vi "Acquisition.vi"() -> ()   [LabVIEW 2018]
uses:
  Type/_Run State.ctl
  Type/_File Type.ctl
  Type/_RT Command.ctl
  Type/_Data Operation.ctl
  Type/_Run Module.ctl
  Configuration/_Global Configuration.vi
  <vilib>/Utility/config.llb/Read Key (Path).vi
  <vilib>/Utility/config.llb/Read Key (String).vi
  <vilib>/Utility/config.llb/Write Key (Path).vi
  <vilib>/Utility/config.llb/Write Key (String).vi
  <vilib>/Utility/file.llb/Read From Spreadsheet File (string).vi
  <vilib>/Utility/miscctls.llb/LVRectTypeDef.ctl
  <vilib>/Utility/config.llb/NI_LVConfig.lvlib
panel:
  in  "Equilibration Time":u32
  in  "Editor":bool
  out "# of Samp":i32=1 caption="# of Samples"
  in  "Sample Description":string
  in  "Sync Mode":enum32{"Manual", "LC Sync"}(radio)
  in  "Data Folder":path
  in  "Save":bool
  in  "Load":bool
  in  "Insert":bool
  in  "Delete":bool
  in  "Import":bool
  in  "Export":bool
  in  "Sample List":i32(listbox)
  in  "Run":bool
  in  "Cancel":bool
  in  "List File":path
  out "Run Time":i32=1 caption="Run Time (ms)"
  in  "Current Sample":i32=1 min=0
  in  "Method File":path
  # "(mS)"
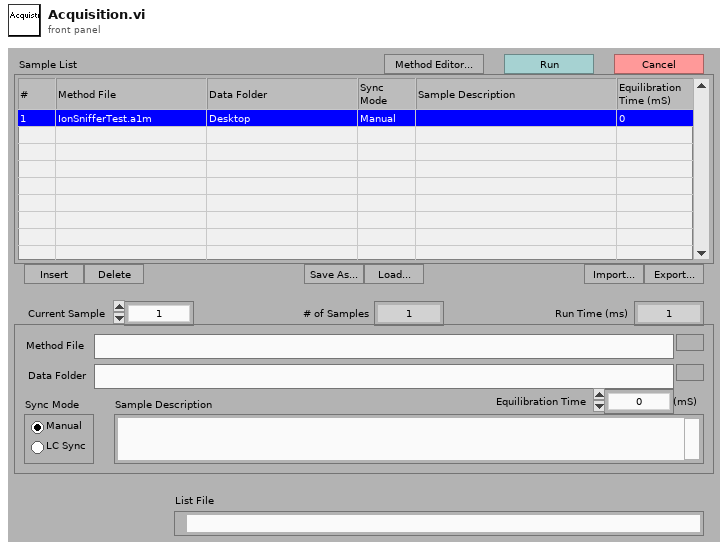
[diagram p1: front panel]
types:
  T1 = typedef "_Run State.ctl" = enum16{"Init", "Update", "Start", "End", "Error"}
  T2 = typedef "_File Type.ctl" = enum16{"Configuration", "Old Configuration", "Calibration", "Resolution", "Diagnostic Method", "Old Method", "Acq Method", "Samp List"}
  T3 = typedef "LVRectTypeDef.ctl" = cluster{"Left":i16, "Top":i16, "Right":i16, "Bottom":i16}
  T4 = typedef "_RT Command.ctl" = enum16{"xml Start Run", "xml Start Actual Run", "xml Stop Run", "xml Runtime Update", "xml Get Status", "xml Get Table", "xml Set Table", "xml Get Configuration", "xml System Status", "xml Set LC Input Logic", "xml Get Data", "xml Get Info", "Start", "StartActualRun", "Stop", "Runtime Update", "Get Data", "Get Info", "Get Status", "Get Param", "Get Config", "Get Table", "Read ADC", "Set Oscillator", "Update Config", "Update Table", "Set All Pol", "Set Pol and DC", "Set Max Mass", "Toggle RP", "Toggle EL", "Set PIC", "Initialize Turbo", "Send Turbo Comm", "Close Turbo", "P1", "P2", "P3", "Send Serial", "Set LC Out", "Get LC In", "Read VAC", "Test Table", "Toggle Power", "Get Startup", "Set Startup", "Get ADC Table", "Set ADC Table", "Get Brief Status", "Get Detail Status", "Auxiliary Update", "Set CC Logics", "Set CC Input Logics", "Ignore Error", "invalid"}
  T5 = typedef "_Data Operation.ctl" = enum8{"Initialize", "Get Data", "Set Data", "Close"}
  T6 = enum32{"Bad", "Idle", "Run top level", "Running"}
  T7 = enum32{"existing file", "new file", "new or existing file", "existing dir", "new dir", "new or existing dir", "existing file (use LLBs)", "new file (use LLBs)", "new or existing file (use LLBs)", "new or existing file or directory (use LLBs)"}
  T8 = typedef "NI_LVConfig.lvlib/Config Data RefNum.ctl" = refnum<k1>
  T9 = cluster{"Update":bool, "Running":bool, "List File":path, "Sample List":string[][]}
  T10 = typedef "_Run Module.ctl" = u16
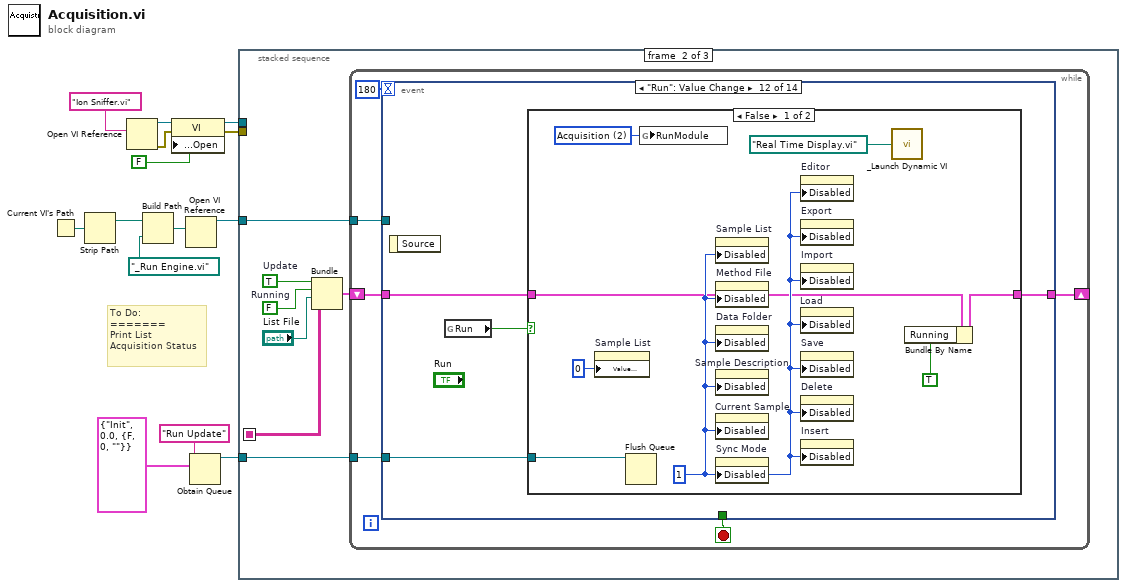
[diagram p0: block diagram]
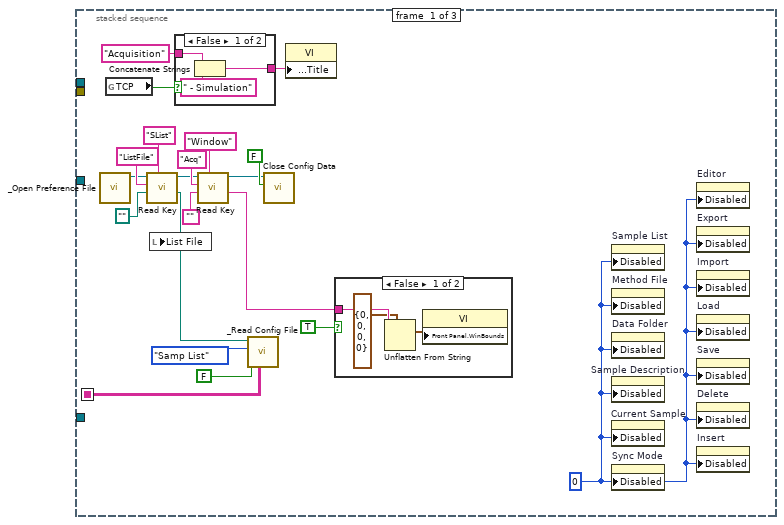
[diagram p2: hidden frame]
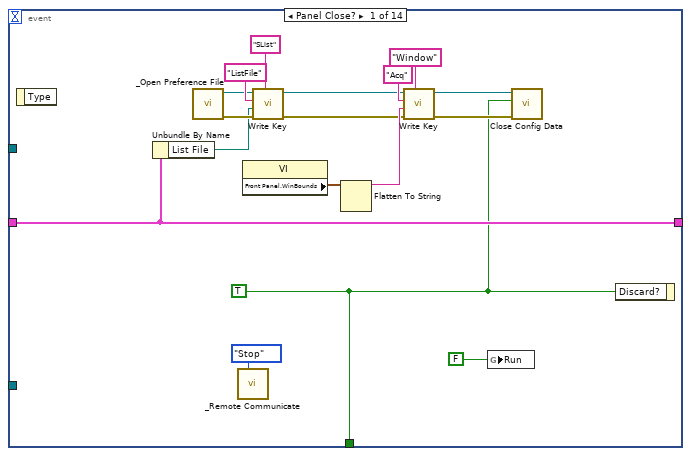
[diagram p5: hidden frame]
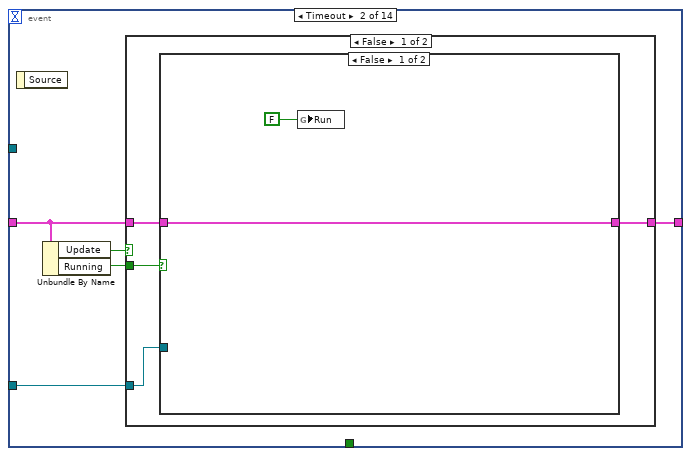
[diagram p6: hidden frame]
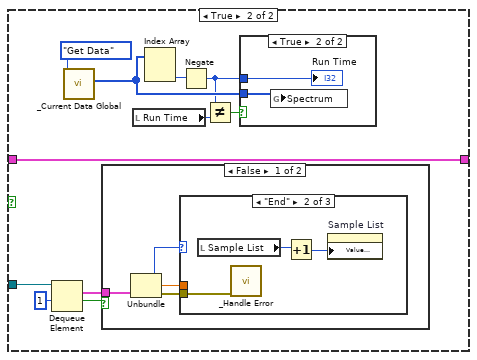
[diagram p7: hidden frame]
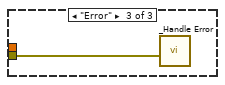
[diagram p10: hidden frame]
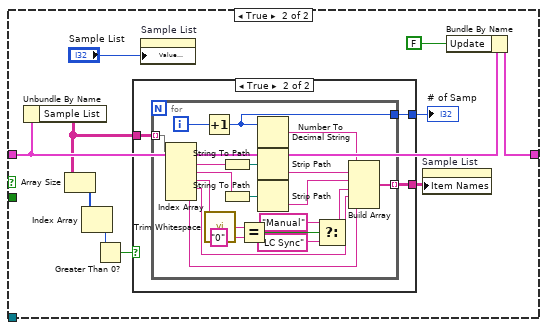
[diagram p12: hidden frame]
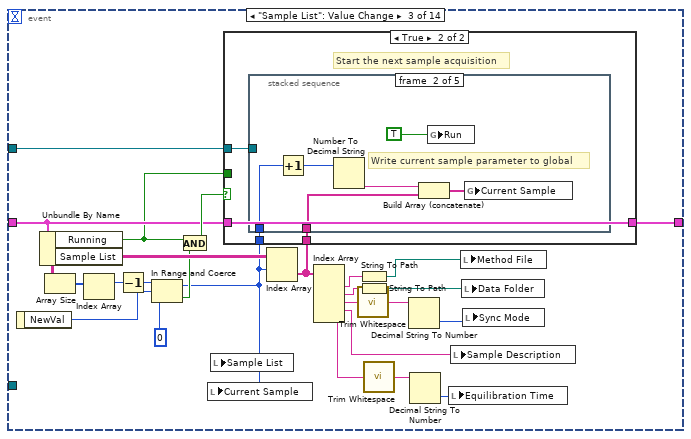
[diagram p14: hidden frame]
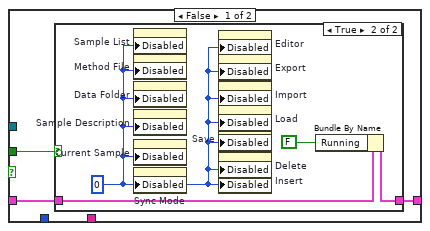
[diagram p15: hidden frame]
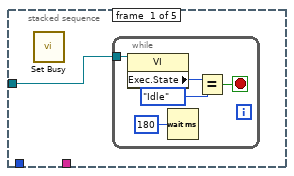
[diagram p17: hidden frame]
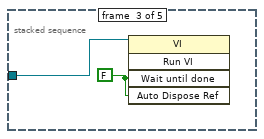
[diagram p18: hidden frame]
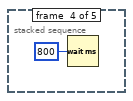
[diagram p19: hidden frame]
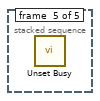
[diagram p20: hidden frame]
diagram:
  # "To Do:\n=======\nPrint List\nAcquisition Status"
  n1 = Current VI's Path() -> (path=w11:path)
  n2 = Strip Path(path=w11) -> (stripped path=w7:path)  [unwired: 1 out]
  n3 = Open VI Reference(vi path="Ion Sniffer.vi") -> (vi reference=w5:refnum<vi>, error out=w4:errorcluster)  [unwired: 1 in, 4 out]
  n4 = Build Path(base path=w7, name or relative path=path "_Run Engine.vi") -> (appended path=w9:path)
  n5 = property class="VI"(reference=w5, error in=w4, "Front Panel Window:Open"=FALSE) -> (reference out=w2:refnum<vi>, error out=w1:errorcluster)
  n6 = Open VI Reference(vi path=w9) -> (vi reference=w8:refnum<vi>)  [unwired: 1 in, 5 out]
  n7 = Obtain Queue(name (unnamed)="Run Update", element data type=cluster{T1, dbl, "error out":errorcluster} {enum."Init", 0.0, "error out"={"status"=FALSE, "code"=0, "source"=""}}) -> (queue out=w12:refnum<queue>)  [unwired: 3 in, 2 out]
  n8 = stacked-sequence {
    seq-local: [w17 _ _] -> [_ w42 _]
    tunnel: w12 -> [_ w48 w344]
    tunnel: w8 -> [_ w47 w343]
    tunnel: w2 -> [_ _ w339]
    tunnel: w1 -> [_ _ w338]
    frame #0 {
      w16 = u8 0 ("Disabled")
      n9 = call "_Open Preference File.vi"() -> ("refnum"=w22:T8)  [unwired: 3 in, 4 out]
      n10 = global read "_Global Configuration.vi" "TCP"() -> (w32:bool)
      n11 = call-poly <vilib>:"Read Key.vi"("section"="SList", "default value"=path "", "key"="ListFile", "refnum"=w22) -> ("value"=w18:path, "refnum out"=w23:T8)  [unwired: 1 in, 5 out]
      n12 = local write "List File"(w18) -> ()
      n13 = case shown="False" w32 {
        tunnel: "Acquisition" ("string") -> [w40 w41]
        tunnel: [w38 w41] -> w33
        frame False {
          n14 = Concatenate Strings(w40, " - Simulation" ("string")) -> (w38:string)
        }
        frame True {
        }
      }
      n15 = call-poly <vilib>:"Read Key.vi"("section"="Window", "default value"="", "key"="Acq" ("section"), "refnum"=w23) -> ("value"=w25:string, "refnum out"=w21:T8)  [unwired: 2 in, 4 out]
      n16 = call "_Read Config File.vi"("advisory dialog? (display:T)"=FALSE, "File Type (config)"=_File_Type."Samp List", "start path  (Not A Path)"=w18) -> ("Sample List"=w17:string[][])  [unwired: 8 out]
      n17 = call <vilib>:"Close Config Data.vi"("write file if changed (T)"=FALSE ("write configuration file? (F)"), "refnum"=w21) -> ()  [unwired: 1 in, 9 out]
      n18 = property class="VI"("Front Panel Window:Title"=w33) -> ()  [unwired: 2 in, 2 out]
      n19 = case shown="False" TRUE {
        tunnel: w25 -> [w37 _]
        frame False {
          n20 = Unflatten From String(type=T3 {"Left"=0, "Top"=0, "Right"=0, "Bottom"=0} ("Front Panel Window:Window Bounds"), binary string=w37) -> (value=w35:T3)  [unwired: 1 in, 4 out]
          n21 = property class="VI"("Front Panel.WinBounds"=w35) -> ()  [unwired: 2 in, 2 out]
        }
        frame True {
        }
      }
      n22 = property on="Sample List" class="MCListbox (strict)"("Disabled"=w16) -> ()  [unwired: 2 in, 2 out]
      n23 = property on="Method File" class="Path"("Disabled"=w16) -> ()  [unwired: 2 in, 2 out]
      n24 = property on="Data Folder" class="Path"("Disabled"=w16) -> ()  [unwired: 2 in, 2 out]
      n25 = property on="Sample Description" class="Str"("Disabled"=w16) -> ()  [unwired: 2 in, 2 out]
      n26 = property on="Current Sample" class="DigNum (strict)"("Disabled"=w16) -> ()  [unwired: 2 in, 2 out]
      n27 = property on="Sync Mode" class="RadioBtnsControl (strict)"("Disabled"=w16) -> ()  [unwired: 2 in, 2 out]
      n28 = property on="Editor" class="Bool"("Disabled"=w16) -> ()  [unwired: 2 in, 2 out]
      n29 = property on="Export" class="Bool"("Disabled"=w16) -> ()  [unwired: 2 in, 2 out]
      n30 = property on="Import" class="Bool"("Disabled"=w16) -> ()  [unwired: 2 in, 2 out]
      n31 = property on="Load" class="Bool"("Disabled"=w16) -> ()  [unwired: 2 in, 2 out]
      n32 = property on="Save" class="Bool"("Disabled"=w16) -> ()  [unwired: 2 in, 2 out]
      n33 = property on="Delete" class="Bool"("Disabled"=w16) -> ()  [unwired: 2 in, 2 out]
      n34 = property on="Insert" class="Bool"("Disabled"=w16) -> ()  [unwired: 2 in, 2 out]
    }
    frame #1 {
      w45 = FALSE  # Running
      w46 = TRUE  # Update
      n35 = Bundle("Update"=w46, "Running"=w45, "List File"="List File", "Sample List"=w42) -> (w44:T9)  [unwired: 1 out]
      n36 = while {
        shift-right: [w51] -> _
        shift-left: w44 -> [w53]
        tunnel: w48 -> [w50]
        tunnel: w47 -> [w49]
        stop <- w54 stop-if-true
        n37 = event shown="[11] \"Run\": Value Change" {
          selector: _ -> [_ _ _ _ _ _ _ _ _ _ _ _ _ _]
          dyn-events: _ -> [_ _ _ _ _ _ _ _ _ _ _ _ _ _]
          timeout: 180 -> [_ _ _ _ _ _ _ _ _ _ _ _ _ _]
          tunnel: [w55 _ _ _ _ _ _ _ _ _ _ _ _ _] -> w54
          tunnel: w53 -> [w66 w74 w144 w190 w206 w219 w227 w241 w249 w269 w305 w309 w325 w337]
          tunnel: [w66 w76 w143 w190 w205 w217 w225 w239 w248 w269 w307 w310 w321 w337] -> w51
          tunnel: w50 -> [_ w75 _ _ _ _ _ _ _ _ _ w311 _ _]
          tunnel: w49 -> [_ _ w145 _ _ _ _ _ _ _ _ _ w324 _]
          event Panel Close? {
            w55 = TRUE ("Discard?")
            n38 = event-data() -> ()  [unwired: 2 out]
            n39 = Unbundle By Name(w66) -> ("List File"=w65:path)
            n40 = call "_Open Preference File.vi"() -> ("error"=w68:errorcluster, "refnum"=w69:T8)  [unwired: 3 in, 3 out]
            n41 = call "_Remote Communicate.vi"("Command"=_RT_Command."Stop") -> ()  [unwired: 5 in, 4 out]
            n42 = property class="VI"() -> ("Front Panel.WinBounds"=w63:T3)  [unwired: 2 in, 2 out]
            n43 = call-poly <vilib>:"Write Key.vi"("section"="SList", "error in (no error)"=w68, "value"=w65, "key"="ListFile", "refnum"=w69) -> ("error out"=w56:errorcluster, "refnum out"=w57:T8)  [unwired: 5 out]
            n44 = Flatten To String(anything=w63) -> (data string=w62:string)  [unwired: 1 in, 4 out]
            n45 = call-poly <vilib>:"Write Key.vi"("section"="Window", "error in (no error)"=w56, "value"=w62, "key"="Acq" ("section"), "refnum"=w57) -> ("error out"=w58:errorcluster, "refnum out"=w59:T8)  [unwired: 1 in, 4 out]
            n46 = global write "_Global Configuration.vi" "Run"(FALSE ("Update")) -> ()
            n47 = call <vilib>:"Close Config Data.vi"("error in (no error)"=w58, "write file if changed (T)"=w55, "refnum"=w59) -> ()  [unwired: 9 out]
            n48 = event-data("Discard?"=w55) -> ()  [unwired: 1 in, 1 out]
          }
          event Timeout {
            n49 = event-data() -> ()  [unwired: 2 out]
            n50 = Unbundle By Name(w74) -> ("Update"=w73:bool, "Running"=w72:bool)
            n51 = case shown="False" w73 {
              tunnel: w74 -> [w78 w113]
              tunnel: [w77 w111] -> w76
              tunnel: w72 -> [w80 _]
              tunnel: w75 -> [w79 _]
              frame False {
                n52 = case shown="False" w80 {
                  tunnel: w79 -> [_ w93]
                  tunnel: w78 -> [w82 w83]
                  tunnel: [w82 w83] -> w77
                  frame False {
                    n53 = global write "_Global Configuration.vi" "Run"(FALSE ("Update")) -> ()
                  }
                  frame True {
                    n54 = Dequeue Element(queue=w93, timeout in ms (-1)=1) -> (element=w91:cluster{T1, dbl, "error out":errorcluster}, timed out?=w90:bool)  [unwired: 1 in, 2 out]
                    n55 = call "_Current Data Global.vi"("Operation"=_Data_Operation."Get Data") -> ("Latest Raw Data"=w86:i32[])  [unwired: 3 in, 3 out]
                    n56 = case shown="False" w90 {
                      tunnel: w91 -> [w99 _]
                      frame False {
                        n57 = Unbundle(w99) -> (w98:T1, w96:dbl, "error out"=w97:errorcluster)
                        n58 = case shown="\"End\"" w98 {
                          tunnel: w97 -> [_ w102 w103]
                          tunnel: w96 -> [_ _ _]
                          frame "Init", Default {
                          }
                          frame "End" {
                            n59 = local read "Sample List"() -> (w101:i32)
                            n60 = call "_Handle Error.vi"("error in (no error)"=w102) -> ()  [unwired: 2 in, 5 out]
                            n61 = Increment(x=w101) -> (x+1=w100:i32)
                            n62 = property on="Sample List" class="MCListbox (strict)"("Value (Signaling)"=w100) -> ()  [unwired: 2 in, 2 out]
                          }
                          frame "Error" {
                            n63 = call "_Handle Error.vi"("error in (no error)"=w103) -> ()  [unwired: 2 in, 5 out]
                          }
                        }
                      }
                      frame True {
                      }
                    }
                    n64 = local read "Run Time"() -> (w88:i32)
                    n65 = Index Array(array=w86) -> (element #2=w85:i32)  [unwired: 2 in, 1 out]
                    n66 = Negate(x=w85) -> (-x=w84:i32)
                    n67 = Not Equal?(x=w84, y=w88) -> (x != y?=w87:bool)
                    n68 = case shown="True" w87 {
                      tunnel: w86 -> [_ w94]
                      tunnel: w84 -> [_ w95]
                      frame False {
                      }
                      frame True {
                        n69 = global write "_Global Configuration.vi" "Spectrum"(w94) -> ()
                        "Run Time" <- w95
                      }
                    }
                  }
                }
              }
              frame True {
                n70 = Unbundle By Name(w113) -> ("Sample List"=w107:string[][])
                n71 = Array Size(array=w107) -> (size(s)=w106:i32[])
                n72 = Index Array(array=w106) -> (element=w105:i32)  [unwired: 1 in]
                n73 = Greater Than 0?(x=w105) -> (x > 0?=w104:bool)
                n74 = case shown="True" w104 {
                  tunnel: [_ w116] -> w109
                  tunnel: [_ w115] -> w108
                  tunnel: w107 -> [_ w114]
                  frame False {
                  }
                  frame True {
                    n75 = for {
                      tunnel: w114 -> [w136] mode=indexing
                      tunnel: [w134] -> w116
                      tunnel: [w119] -> w115 mode=indexing
                      i -> [w135]
                      n76 = Index Array(array=w136) -> (element #1=w133:string, element #2=w130:string, element #3=w129:string, element #4=w120:string, element #5=w117:string)  [unwired: 5 in]
                      n77 = Increment(x=w135) -> (x+1=w134:i32)
                      n78 = call <vilib>:"Trim Whitespace.vi"("string"=w129) -> ("trimmed string"=w127:string)  [unwired: 1 in]
                      n79 = String To Path(string=w133) -> (path=w132:path)
                      n80 = String To Path(string=w130) -> (path=w131:path)
                      n81 = Equal?(x=w127, y="0") -> (x = y?=w128:bool)
                      n82 = Number To Decimal String(number=w134) -> (decimal integer string=w124:string)  [unwired: 1 out]
                      n83 = Strip Path(path=w132) -> (name=w123:string)  [unwired: 1 out]
                      n84 = Strip Path(path=w131) -> (name=w122:string)  [unwired: 1 out]
                      n85 = Select(t="Manual" ("y"), s=w128, f="LC Sync" ("y")) -> (s? t:f=w121:string)
                      n86 = Build Array(w124, w123, w122, w121, w120, w117) -> (w119:string[])
                    }
                  }
                }
                "# of Samp" <- w109
                n87 = property on="Sample List" class="MCListbox (strict)"("Value (Signaling)"="Sample List") -> ()  [unwired: 2 in, 2 out]
                n88 = property on="Sample List" class="MCListbox (strict)"("Item Names"=w108) -> ()  [unwired: 2 in, 2 out]
                n89 = Bundle By Name(cluster=w113, "Update"=FALSE) -> (w111:T9)
              }
            }
          }
          event "Sample List": Value Change {
            n90 = event-data() -> ("NewVal"=w161:i32)  [unwired: 1 out]
            n91 = Unbundle By Name(w144) -> ("Running"=w142:bool, "Sample List"=w158:string[][])
            n92 = Array Size(array=w158) -> (size(s)=w156:i32[])
            n93 = Index Array(array=w156) -> (element=w157:i32)  [unwired: 1 in]
            n94 = Decrement(x=w157) -> (x-1=w159:i32)
            n95 = In Range and Coerce(upper limit=w159, x=w161, lower limit=0) -> (coerced(x)=w140:i32, In Range?=w147:bool)
            n96 = And(x=w142, y=w147) -> (x .and. y?=w146:bool)
            n97 = local write "Current Sample"(w140) -> ()
            n98 = local write "Sample List"(w140) -> ()
            n99 = Index Array(array=w158, index (row)=w140) -> (element=w141:string[])  [unwired: 1 in]
            n100 = case shown="True" w146 {
              tunnel: w145 -> [_ w173]
              tunnel: w144 -> [w164 w172]
              tunnel: [w163 w172] -> w143
              tunnel: w142 -> [w162 _]
              tunnel: w141 -> [_ w171]
              tunnel: w140 -> [_ w170]
              frame False {
                n101 = case shown="True" w162 {
                  tunnel: w164 -> [w165 w169]
                  tunnel: [w165 w168] -> w163
                  frame False {
                  }
                  frame True {
                    w167 = u8 0 ("Disabled")
                    n102 = property on="Sample List" class="MCListbox (strict)"("Disabled"=w167) -> ()  [unwired: 2 in, 2 out]
                    n103 = property on="Method File" class="Path"("Disabled"=w167) -> ()  [unwired: 2 in, 2 out]
                    n104 = property on="Data Folder" class="Path"("Disabled"=w167) -> ()  [unwired: 2 in, 2 out]
                    n105 = property on="Sample Description" class="Str"("Disabled"=w167) -> ()  [unwired: 2 in, 2 out]
                    n106 = property on="Current Sample" class="DigNum (strict)"("Disabled"=w167) -> ()  [unwired: 2 in, 2 out]
                    n107 = property on="Sync Mode" class="RadioBtnsControl (strict)"("Disabled"=w167) -> ()  [unwired: 2 in, 2 out]
                    n108 = property on="Editor" class="Bool"("Disabled"=w167) -> ()  [unwired: 2 in, 2 out]
                    n109 = property on="Export" class="Bool"("Disabled"=w167) -> ()  [unwired: 2 in, 2 out]
                    n110 = property on="Import" class="Bool"("Disabled"=w167) -> ()  [unwired: 2 in, 2 out]
                    n111 = property on="Load" class="Bool"("Disabled"=w167) -> ()  [unwired: 2 in, 2 out]
                    n112 = property on="Save" class="Bool"("Disabled"=w167) -> ()  [unwired: 2 in, 2 out]
                    n113 = property on="Delete" class="Bool"("Disabled"=w167) -> ()  [unwired: 2 in, 2 out]
                    n114 = property on="Insert" class="Bool"("Disabled"=w167) -> ()  [unwired: 2 in, 2 out]
                    n115 = Bundle By Name(cluster=w169, "Running"=FALSE) -> (w168:T9)
                  }
                }
              }
              frame True {
                # "Start the next sample acquisition"
                n116 = stacked-sequence {
                  tunnel: w173 -> [w174 _ w186 _ _]
                  tunnel: w171 -> [_ w184 _ _ _]
                  tunnel: w170 -> [_ w181 _ _ _]
                  frame #0 {
                    n117 = call <vilib>:"Set Busy.vi"() -> ()  [unwired: 4 in, 8 out]
                    n118 = while {
                      tunnel: w174 -> [w179]
                      stop <- w176 stop-if-true
                      n119 = property class="VI"(reference=w179) -> ("Exec.State"=w178:T6)  [unwired: 1 in, 2 out]
                      n120 = Wait (ms)(milliseconds to wait=u32 180) -> ()  [unwired: 1 out]
                      n121 = Equal?(x=w178, y=T6."Idle") -> (x = y?=w176:bool)
                    }
                  }
                  frame #1 {
                    # "Write current sample parameter to global"
                    n122 = Increment(x=w181) -> (x+1=w180:i32)
                    n123 = Number To Decimal String(number=w180) -> (decimal integer string=w182:string)  [unwired: 1 out]
                    n124 = Build Array (concatenate)(w182, w184) -> (w183:string[])
                    n125 = global write "_Global Configuration.vi" "Run"(TRUE ("Update")) -> ()
                    n126 = global write "_Global Configuration.vi" "Current Sample"(w183) -> ()
                  }
                  frame #2 {
                    w187 = FALSE ("Wait until done")
                    n127 = invoke class="VI" method="Run VI"(reference=w186, "Wait until done"=w187, "Auto Dispose Ref"=w187) -> ()  [unwired: 2 in, 5 out]
                  }
                  frame #3 {
                    n128 = Wait (ms)(milliseconds to wait=u32 800) -> ()  [unwired: 1 out]
                  }
                  frame #4 {
                    n129 = call <vilib>:"Unset Busy.vi"() -> ()  [unwired: 2 in, 10 out]
                  }
                }
              }
            }
            n130 = Index Array(array=w141) -> (element #1=w152:string, element #2=w153:string, element #3=w154:string, element #4=w155:string, element #5=w138:string)  [unwired: 5 in]
            n131 = call <vilib>:"Trim Whitespace.vi"("string"=w154) -> ("trimmed string"=w149:string)  [unwired: 1 in]
            n132 = String To Path(string=w152) -> (path=w151:path)
            n133 = String To Path(string=w153) -> (path=w150:path)
            n134 = call <vilib>:"Trim Whitespace.vi"("string"=w138) -> ("trimmed string"=w139:string)  [unwired: 1 in]
            n135 = Decimal String To Number(string=w149) -> (number=w148:i32)  [unwired: 3 out]
            n136 = Decimal String To Number(string=w139) -> (number=w137:i32)  [unwired: 3 out]
            n137 = local write "Equilibration Time"(w137) -> ()
            n138 = local write "Sample Description"(w155) -> ()
            n139 = local write "Method File"(w151) -> ()
            n140 = local write "Data Folder"(w150) -> ()
            n141 = local write "Sync Mode"(w148) -> ()
          }
          event "Current Sample": Value Change {
            n142 = event-data() -> ("NewVal"=w189:i32)  [unwired: 1 out]
            n143 = property on="Sample List" class="MCListbox (strict)"("Value (Signaling)"=w189) -> ()  [unwired: 2 in, 2 out]
          }
          event "Insert": Value Change {
            n144 = event-data() -> ()  [unwired: 2 out]
            n145 = call "Please enter # of samples to insert."() -> ("# of Samples to Insert"=w203:dbl)  [unwired: 2 in, 17 out]
            n146 = Unbundle By Name(w206) -> ("Sample List"=w198:string[][])
            n147 = local read "Sample List"() -> (w197:i32)
            n148 = To Long Integer(number=w203) -> (32bit integer=w202:i32)
            n149 = In Range and Coerce(upper limit=2147483647, x=w202, lower limit=1) -> (coerced(x)=w199:i32)  [unwired: 1 out]
            n150 = Index Array(array=w198, index (row)=w197) -> (element=w193:string[])  [unwired: 1 in]
            n151 = Array Size(array=w193) -> (size(s)=w195:i32)
            n152 = Greater Than 0?(x=w195) -> (x > 0?=w194:bool)
            n153 = Select(t=w193, s=w194, f=string[] ["", "", "1", "", "0"] ("appended array")) -> (s? t:f=w191:string[])
            n154 = for {
              N: w199 -> [_]
              shift-right: [w208] -> w196
              shift-left: w198 -> [w210]
              tunnel: w197 -> [w209]
              tunnel: w191 -> [w207]
              n155 = Insert Into Array(array=w210, index (row)=w209, new element=w207) -> (w208:string[][])  [unwired: 1 in]
            }
            n156 = Bundle By Name(cluster=w206, "Sample List"=w196, "Update"=TRUE) -> (w205:T9)
          }
          event "Delete": Value Change {
            n157 = event-data() -> ()  [unwired: 2 out]
            n158 = Unbundle By Name(w219) -> ("Sample List"=w218:string[][])
            n159 = Two Button Dialog(message="Please choose a delete option.", 1:"Delete All Samples" ("T button name (\"OK\")"), 2:"Delete Current Sample" ("T button name (\"OK\")")) -> (T button?=w211:bool)
            n160 = case shown="True" w211 {
              tunnel: w218 -> [_ w223]
              tunnel: [_ w220] -> w216
              frame False {
              }
              frame True {
                n161 = local read "Sample List"() -> (w221:i32)
                n162 = Delete From Array(array=w223, length=1, index (row)=w221) -> (array with subset deleted=w220:string[][])  [unwired: 1 in, 1 out]
              }
            }
            n163 = Bundle By Name(cluster=w219, "Sample List"=w216, "Update"=TRUE) -> (w217:T9)
          }
          event "Save": Value Change {
            n164 = event-data() -> ()  [unwired: 2 out]
            n165 = Unbundle By Name(w227) -> ("List File"=w229:path, "Sample List"=w228:string[][])
            n166 = call "_Save Config File.vi"("Sample List"=w228, "File Type (config)"=_File_Type."Samp List", "start path  (Not A Path)"=w229) -> ("error"=w226:bool, "new file path"=w224:path)  [unwired: 5 in, 2 out]
            n167 = case shown="False" w226 {
              tunnel: w227 -> [w233 w234]
              tunnel: [w232 w234] -> w225
              tunnel: w224 -> [w231 _]
              frame False {
                n168 = local write "List File"(w231) -> ()
                n169 = Bundle By Name(cluster=w233, "List File"=w231) -> (w232:T9)
              }
              frame True {
              }
            }
          }
          event "Load": Value Change {
            n170 = event-data() -> ()  [unwired: 2 out]
            n171 = Unbundle By Name(w241) -> ("List File"=w238:path)
            n172 = call "_Read Config File.vi"("File Type (config)"=_File_Type."Samp List", "start path  (Not A Path)"=w238) -> ("error"=w240:bool, "new file path"=w235:path, "Sample List"=w236:string[][])  [unwired: 3 in, 4 out]
            n173 = case shown="False" w240 {
              tunnel: w241 -> [w246 w247]
              tunnel: [w245 w247] -> w239
              tunnel: w235 -> [w244 _]
              tunnel: w236 -> [w242 _]
              frame False {
                n174 = Bundle By Name(cluster=w246, "Update"=TRUE, "Sample List"=w242, "List File"=w244) -> (w245:T9)
                n175 = local write "List File"(w244) -> ()
              }
              frame True {
              }
            }
          }
          event "Import": Value Change {
            n176 = event-data() -> ()  [unwired: 2 out]
            n177 = Unbundle By Name(w249) -> ("List File"=w252:path)
            n178 = call "_Get File.vi"("For Write (T)"=FALSE, "select mode (new or existing)"=T7."existing file", "extension (isd)"="*.txt" ("pattern (all files)"), "prompt"="Please select a sample list import file.", "Start Path"=w252) -> ("Seleted File"=w250:path, "Exists"=w258:bool, "Succeeded"=w257:bool)  [unwired: 1 in, 1 out]
            n179 = And(x=w257, y=w258) -> (x .and. y?=w251:bool)
            n180 = case shown="True" w251 {
              tunnel: w250 -> [_ w264]
              tunnel: w249 -> [w259 w263]
              tunnel: [w259 w262] -> w248
              frame False {
              }
              frame True {
                n181 = call-poly <vilib>:"Read From Spreadsheet File.vi"("file path (dialog if empty)"=w264) -> ("all rows"=w266:string[][])  [unwired: 3 in, 7 out]
                n182 = Delete From Array(array=w266, length=1, index (row)=0) -> (array with subset deleted=w261:string[][])  [unwired: 1 in, 1 out]
                n183 = Bundle By Name(cluster=w263, "Update"=TRUE, "Sample List"=w261) -> (w262:T9)
              }
            }
          }
          event "Export": Value Change {
            n184 = event-data() -> ()  [unwired: 2 out]
            n185 = Unbundle By Name(w269) -> ("Sample List"=w270:string[][], "List File"=w277:path)
            n186 = property on="Sample List" class="MCListbox (strict)"() -> ("ColHdrString"=w274:string[])  [unwired: 2 in, 2 out]
            n187 = call "_Get File.vi"("For Write (T)"=TRUE, "select mode (new or existing)"=T7."new or existing file", "default name"="My Sample List", "extension (isd)"="*.txt" ("pattern (all files)"), "prompt"="Please enter a sample list export file name.", "Start Path"=w277) -> ("Seleted File"=w276:path, "Succeeded"=w275:bool)  [unwired: 2 out]
            n188 = Delete From Array(array=w274, length=1, index=0) -> (array with subset deleted=w271:string[])  [unwired: 1 out]
            n189 = case shown="True" w275 {
              tunnel: w276 -> [_ w283]
              tunnel: w271 -> [_ w285]
              tunnel: w270 -> [_ w284]
              frame False {
              }
              frame True {
                n190 = Build Array (concatenate)(w285, w284) -> (w282:string[][])
                n191 = call "_Export Table To Text File.vi"("2D data"=w282, "file path (dialog if empty)"=w283) -> ()  [unwired: 4 in, 3 out]
              }
            }
          }
          event "Method File", "Data Folder", "Sync Mode", "Sample Description", "Equilibration Time": Value Change {
            n192 = event-data() -> ()  [unwired: 2 out]
            n193 = Unbundle By Name(w305) -> ("Sample List"=w293:string[][])
            n194 = Path To String(path="Data Folder") -> (string=w301:string)
            n195 = Path To String(path="Method File") -> (string=w302:string)
            n196 = Index Array(array=w293, index (row)=0) -> (element=w296:string[])  [unwired: 1 in]
            n197 = Number To Decimal String(number="Sync Mode") -> (decimal integer string=w298:string)  [unwired: 1 out]
            n198 = Number To Decimal String(number="Equilibration Time") -> (decimal integer string=w286:string)  [unwired: 1 out]
            n199 = Array Size(array=w296) -> (size(s)=w295:i32)
            n200 = Build Array(w302, w301, w298, "Sample Description", w286) -> (w291:string[])
            n201 = Greater Than 0?(x=w295) -> (x > 0?=w294:bool)
            n202 = Replace Array Subset(array=w293, new element=w291, index (row)="Current Sample") -> (w289:string[][])  [unwired: 1 in]
            n203 = Insert Into Array(array=w293, index (row)="Current Sample", new element=w291) -> (w290:string[][])  [unwired: 1 in]
            n204 = Select(t=w289, s=w294, f=w290) -> (s? t:f=w288:string[][])
            n205 = Bundle By Name(cluster=w305, "Update"=TRUE, "Sample List"=w288) -> (w307:T9)
          }
          event "Run": Value Change {
            n206 = event-data() -> ()  [unwired: 2 out]
            n207 = global read "_Global Configuration.vi" "Run"() -> (w308:bool)
            n208 = case shown="False" w308 {
              tunnel: w311 -> [w319 _]
              tunnel: [w317 w320] -> w310
              tunnel: w309 -> [w312 w320]
              frame False {
                w316 = T10 2 items=["Diagnostics", "Tune", "Acquisition"] ("RunModule")
                w315 = u8 1 ("Disabled")
                n209 = property on="Sample List" class="MCListbox (strict)"("Value (Signaling)"=0) -> ()  [unwired: 2 in, 2 out]
                n210 = Flush Queue(queue=w319) -> ()  [unwired: 1 in, 3 out]
                n211 = global write "_Global Configuration.vi" "RunModule"(w316) -> ()
                n212 = property on="Sample List" class="MCListbox (strict)"("Disabled"=w315) -> ()  [unwired: 2 in, 2 out]
                n213 = property on="Method File" class="Path"("Disabled"=w315) -> ()  [unwired: 2 in, 2 out]
                n214 = property on="Data Folder" class="Path"("Disabled"=w315) -> ()  [unwired: 2 in, 2 out]
                n215 = property on="Sample Description" class="Str"("Disabled"=w315) -> ()  [unwired: 2 in, 2 out]
                n216 = property on="Current Sample" class="DigNum (strict)"("Disabled"=w315) -> ()  [unwired: 2 in, 2 out]
                n217 = property on="Sync Mode" class="RadioBtnsControl (strict)"("Disabled"=w315) -> ()  [unwired: 2 in, 2 out]
                n218 = property on="Editor" class="Bool"("Disabled"=w315) -> ()  [unwired: 2 in, 2 out]
                n219 = property on="Export" class="Bool"("Disabled"=w315) -> ()  [unwired: 2 in, 2 out]
                n220 = property on="Import" class="Bool"("Disabled"=w315) -> ()  [unwired: 2 in, 2 out]
                n221 = property on="Load" class="Bool"("Disabled"=w315) -> ()  [unwired: 2 in, 2 out]
                n222 = property on="Save" class="Bool"("Disabled"=w315) -> ()  [unwired: 2 in, 2 out]
                n223 = property on="Delete" class="Bool"("Disabled"=w315) -> ()  [unwired: 2 in, 2 out]
                n224 = property on="Insert" class="Bool"("Disabled"=w315) -> ()  [unwired: 2 in, 2 out]
                n225 = call "_Launch Dynamic VI.vi"("VI Name"=path "Real Time Display.vi" ("name or relative path")) -> ()  [unwired: 3 in, 1 out]
                n226 = Bundle By Name(cluster=w312, "Running"=TRUE) -> (w317:T9)
              }
              frame True {
              }
            }
          }
          event "Cancel": Value Change {
            n227 = event-data() -> ()  [unwired: 7 out]
            n228 = stacked-sequence {
              tunnel: w325 -> [_ w328 _]
              tunnel: [_ w328 _] -> w322
              tunnel: w324 -> [_ w327 _]
              frame #0 {
                n229 = call <vilib>:"Set Busy.vi"() -> ()  [unwired: 4 in, 8 out]
                n230 = global write "_Global Configuration.vi" "Run"(FALSE ("Update")) -> ()
              }
              frame #1 {
                n231 = while {
                  tunnel: w327 -> [w333]
                  stop <- w330 stop-if-true
                  n232 = property class="VI"(reference=w333) -> ("Exec.State"=w332:T6)  [unwired: 1 in, 2 out]
                  n233 = Wait (ms)(milliseconds to wait=u32 180) -> ()  [unwired: 1 out]
                  n234 = Equal?(x=w332, y=T6."Idle") -> (x = y?=w330:bool)
                }
              }
              frame #2 {
                w335 = u8 0 ("Disabled")
                n235 = call <vilib>:"Unset Busy.vi"() -> ()  [unwired: 2 in, 10 out]
                n236 = call "_Remote Wait Until Done.vi"() -> ("error out"=w334:errorcluster)  [unwired: 2 in, 1 out]
                n237 = call "_Remote Park Lens.vi"("error in"=w334) -> ()  [unwired: 1 in, 6 out]
                n238 = property on="Sample List" class="MCListbox (strict)"("Disabled"=w335) -> ()  [unwired: 2 in, 2 out]
                n239 = property on="Method File" class="Path"("Disabled"=w335) -> ()  [unwired: 2 in, 2 out]
                n240 = property on="Data Folder" class="Path"("Disabled"=w335) -> ()  [unwired: 2 in, 2 out]
                n241 = property on="Sample Description" class="Str"("Disabled"=w335) -> ()  [unwired: 2 in, 2 out]
                n242 = property on="Current Sample" class="DigNum (strict)"("Disabled"=w335) -> ()  [unwired: 2 in, 2 out]
                n243 = property on="Sync Mode" class="RadioBtnsControl (strict)"("Disabled"=w335) -> ()  [unwired: 2 in, 2 out]
                n244 = property on="Editor" class="Bool"("Disabled"=w335) -> ()  [unwired: 2 in, 2 out]
                n245 = property on="Export" class="Bool"("Disabled"=w335) -> ()  [unwired: 2 in, 2 out]
                n246 = property on="Import" class="Bool"("Disabled"=w335) -> ()  [unwired: 2 in, 2 out]
                n247 = property on="Load" class="Bool"("Disabled"=w335) -> ()  [unwired: 2 in, 2 out]
                n248 = property on="Save" class="Bool"("Disabled"=w335) -> ()  [unwired: 2 in, 2 out]
                n249 = property on="Delete" class="Bool"("Disabled"=w335) -> ()  [unwired: 2 in, 2 out]
                n250 = property on="Insert" class="Bool"("Disabled"=w335) -> ()  [unwired: 2 in, 2 out]
              }
            }
            n251 = Bundle By Name(cluster=w322, "Running"=FALSE) -> (w321:T9)
          }
          event "Editor": Value Change {
            n252 = event-data() -> ()  [unwired: 2 out]
            n253 = local read "Method File"() -> (w336:path)
            n254 = call "Method Editor.vi"("Method File:"=w336) -> ()
          }
        }
      }
    }
    frame #2 {
      n255 = property class="VI"(reference=w339, error in=w338, "Front Panel Window:Open"=TRUE) -> (reference out=w340:refnum<vi>, error out=w341:errorcluster)
      n256 = Close Reference(reference=w343) -> ()  [unwired: 1 in, 1 out]
      n257 = Release Queue(queue=w344) -> ()  [unwired: 1 in, 4 out]
      n258 = Close Reference(reference=w340, error in (no error)=w341) -> ()  [unwired: 1 out]
    }
  }
